vi "peekNextLine.vi"(8 "error in":errorcluster, 11 "file* in":refnum<file>) -> (0 "error out":errorcluster, 2 "nextLine":string, 3 "file* out":refnum<file>)   [LabVIEW 2013]
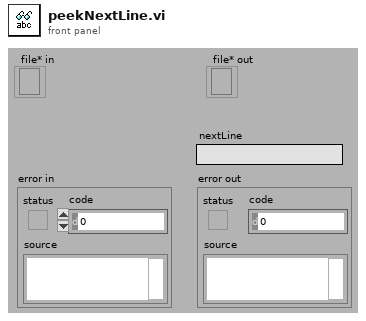
[diagram p1: front panel]
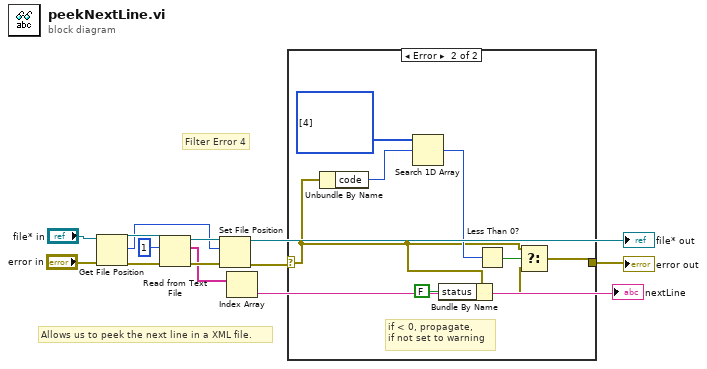
[diagram p0: block diagram]
diagram:
  # "Filter Error 4"
  # "Allows us to peek the next line in a XML file."
  n1 = Get File Position(4:"error in", 7:"file* in") -> (0:w11:errorcluster, 2:w8:i64, 3:w12:refnum<file>)
  n2 = Read from Text File(file (use dialog)=w12, count=1, error in=w11) -> (refnum out=w9:refnum<file>, text=w4:string[], error out=w10:errorcluster)  [unwired: 1 in, 1 out]
  n3 = Set File Position(offset (in bytes) (0)=w8, refnum=w9, error in=w10) -> (refnum out=→"file* out":refnum<file>, error out=w2:errorcluster)  [unwired: 1 in]
  n4 = Index Array(array=w4) -> (element=→"nextLine":string)  [unwired: 1 in]
  n5 = case shown="Error" w2 {
    selector: w2 -> [w14 w18]
    tunnel: [w14 w15] -> w1
    frame No Error {
    }
    frame Error {
      # "if < 0, propagate,\nif not set to warning"
      n6 = Unbundle By Name(w18) -> ("code"=w21:i32)
      n7 = Search 1D Array(1D array=i32[] [4], element=w21) -> (index of element=w20:i32)  [unwired: 1 in]
      n8 = Bundle By Name(cluster=w18, "status"=FALSE) -> (w17:errorcluster)
      n9 = Less Than 0?(x=w20) -> (x < 0?=w19:bool)
      n10 = Select(t=w18, s=w19, f=w17) -> (s? t:f=w15:errorcluster)
    }
  }
  "error out" <- w1
